vi "Card Strength.vi"(11 "Hand In":string) -> (3 "Hand Out":string)   [LabVIEW 2021]
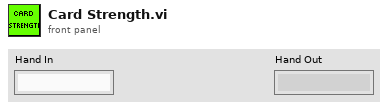
[diagram p1: front panel]
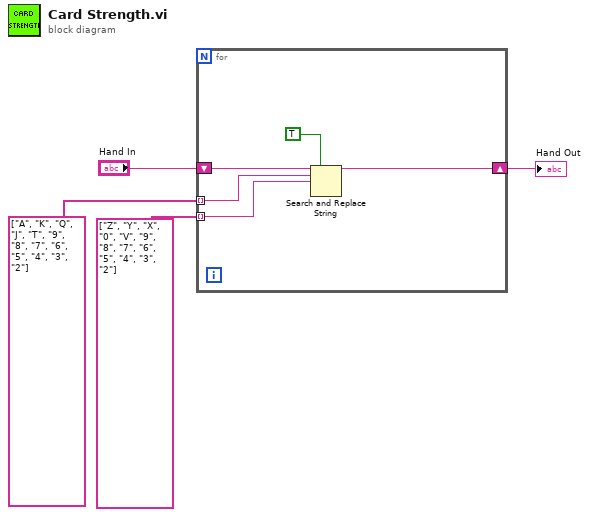
[diagram p0: block diagram]
diagram:
  n1 = for {
    shift-right: [w8] -> w3
    shift-left: "Hand In" -> [w9]
    tunnel: string[] ["A", "K", "Q", "J", "T", "9", "8", "7", "6", "5", "4", "3", "2"] -> [w6] mode=indexing
    tunnel: string[] ["Z", "Y", "X", "0", "V", "9", "8", "7", "6", "5", "4", "3", "2"] -> [w5] mode=indexing
    n2 = Search and Replace String(replace all?=TRUE, input string=w9, search string=w6, replace string=w5) -> (result string=w8:string)  [unwired: 4 in, 3 out]
  }
  "Hand Out" <- w3
